vi "rx.vi"(8 "error in (no error)":errorcluster, 11 "Cluster":T1={"channel"=5180, "channel2"=5290, "rxMode"=0, "rxChain"=1, "wlanMode"=8, "rateMask"=60, "antenna"=0, "bandwidth"=0}) -> (0 "error out":errorcluster)   [LabVIEW 2015, in "QCA_DUT_Func.lvlib"]
uses:
  QCA_DUT_Func.lvlib
  DLLTest.dll
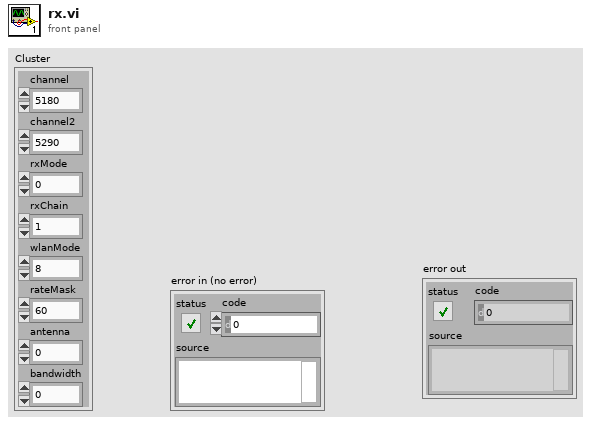
[diagram p1: front panel]
types:
  T1 = cluster{"channel":u32, "channel2":u32, "rxMode":u32, "rxChain":u32, "wlanMode":u32, "rateMask":u32, "antenna":u32, "bandwidth":u32}
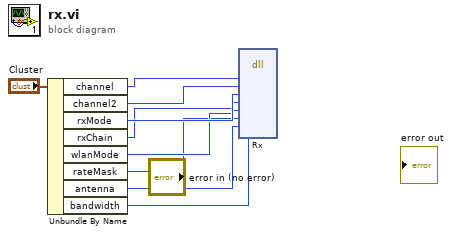
[diagram p0: block diagram]
diagram:
  n1 = Unbundle By Name("Cluster") -> ("channel"=w8:u32, "channel2"=w7:u32, "rxMode"=w6:u32, "rxChain"=w5:u32, "wlanMode"=w4:u32, "rateMask"=w3:u32, "antenna"=w2:u32, "bandwidth"=w1:u32)
  n2 = dll-call lib="D:/Cobham_QCA9984/VI/DLLTest.dll" fn="Rx"("channel"=w8, "channel2"=w7, "rxMode"=w6, "rxChain"=w5, "wlanMode"=w4, "rateMask"=w3, "antenna"=w2, "bandwidth"=w1) -> ()  [unwired: 12 in, 2 out]
